vi "PH_ImageOperator.PC set Position On.vi"(0 "i ref in":refnum<vi>, 2 "Position on":bool, 5 "error in (no error)":errorcluster) -> (14 "i ref out":refnum<vi>, 19 "error out":errorcluster)   [LabVIEW 2014, in "PH_ImageOperator.lvlib"]
doc: "This is the Action of the \"PositionOn\"-Case: It sets some attributes and GUI elements."
uses:
  PH_ImageOperator.lvlib
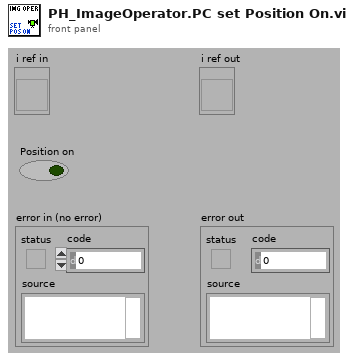
[diagram p1: front panel]
types:
  T1 = typedef "PH_ImageOperator.lvlib/PH_ImageOperator.i attribute.ctl" = cluster{"GUI Refs":cluster{"Delete":refnum<vi>, "Calibration status":refnum<vi>, "BI subtracted":refnum<vi>, "calc Energy":refnum<vi>, "Energy: expected value":refnum<vi>, "Energy: Tolerance":refnum<vi>, "Energy calculated":refnum<vi>, "Energy":refnum<vi>, "calc Beam Anal":refnum<vi>, "Maj Diam 1/esquare":refnum<vi>, "Min Diam 1/esquare":refnum<vi>, "Azi Angle":refnum<vi>, "Min/Maj Diam esquare":refnum<vi>, "Beam analysed":refnum<vi>, "CoG - x":refnum<vi>, "CoG - y":refnum<vi>, "BA: Method":refnum<vi>, "BA: Steps":refnum<vi>, "BA: Factor":refnum<vi>, "calc Traces":refnum<vi>, "Traces: Fit Gauss":refnum<vi>, "Traces calculated":refnum<vi>, "Maj FWHM":refnum<vi>, "Min FWHM":refnum<vi>, "Major Trace":refnum<vi>, "Minor Trace":refnum<vi>, "Maj Fit Order":refnum<vi>, "Min Fit Order":refnum<vi>, "Position calculated":refnum<vi>, "Position":refnum<vi>, "Type":refnum<vi>, "Center":refnum<vi>, "exp - X":refnum<vi>, "exp - Y":refnum<vi>, "Tolerance":refnum<vi>, "f":refnum<vi>, "M":refnum<vi>, "D":refnum<vi>, "q":refnum<vi>, "Dummy Method":refnum<vi>, "Dummy Type":refnum<vi>, "Global On":refnum<vi>, "Traces: No offset":refnum<vi>, "Maj 99%":refnum<vi>, "Min 99%":refnum<vi>, "GUI FF Image":refnum<vi>, "calc Fill Factor":refnum<vi>, "FF calculated":refnum<vi>, "Fill Factor: Filter?":refnum<vi>, "FF: Damage Threshold":refnum<vi>, "FF: Threshold":refnum<vi>, "FF: max allow. Energy":refnum<vi>, "FF: Fillfactor":refnum<vi>, "Calibration data":refnum<vi>}, "List of GUIs":string[], "Calibration":cluster{"Status":T2, "Calibration data":T3, "Calibration Data File":path}, "Final Image":cluster{"BI Subtraction Failure":bool}, "Energy":cluster{"on":bool, "expected value [mJ]":dbl, "Tolerance [%]":dbl, "State":T2, "Energy [mJ]":dbl, "Unit":string, "calculated @":timestamp}, "Beam Analysis":cluster{"on":bool, "Data":T4, "Method":bool, "Steps":i32, "Factor":i32, "ROI":cluster{"Left":i32, "Top":i32, "Right":i32, "Bottom":i32}, "analysed @":timestamp}, "Trace Analysis":cluster{"on":bool, "Fit on":bool, "Maj FWHM":dbl, "Min FWHM":dbl, "Maj Fit Order":i32, "Min Fit Order":i32, "No Offset":bool, "Maj 99%":dbl, "Min 99%":dbl, "Traces":cluster{"XScaleName":string, "Y Scale Minimum":sgl, "Y Scale Maximum":sgl, "X Scale Minimum":sgl, "X Scale Maximum":sgl, "Traces":cluster{"Index":sgl[], "Trace":dbl[]}[]}[], "analysed @":timestamp}, "Position Analysis":cluster{"on":bool, "exp - X":i32, "exp - Y":i32, "focal length [mm]":dbl, "Magnification":dbl, "Delta":dbl, "Theta":dbl, "Tolerance":dbl, "Type":bool, "analysed @":timestamp}, "Fill Factor":cluster{"on":bool, "Filter on?":bool, "Threshold":dbl, "Damage Threshold [J/cm²]":dbl, "Fillfactor":dbl, "Max. allowed Energy [J]":dbl, "calculated @":timestamp}, "Statistician Service ID":i32, "Images":cluster{"Background":T5, "OP":T5, "GUI":T5, "BA: ROI":T5, "Trace: Turn":T5, "FF: Main":T5, "FF: Help":T5, "PSDB: BG":T5, "PSDB: OP":T5, "PSDB: FF":T5}}
  T2 = typedef "PH_StatusHandler.lvlib/PH_StatusHandler.Status.ctl" = i16
  T3 = typedef "PH_ImageCalibrator.lvlib/PH_ImageCalibrator.Calibration Data.ctl" = cluster{"Date":string, "Time":string, "Cam Settings":cluster{"Cam ID":string, "Gain":dbl, "Brightness":dbl, "Shutter":dbl, "Cam Error":bool, "Mode":i32}, "Background Image":cluster{"Image":dbl[][], "Image Error":bool}, "Linear Calibration":cluster{"Calibration Factor":dbl, "not mm or mrad":bool}, "Energy Calibration":cluster{"Calibration Factor":dbl, "no mJ":bool}}
  T4 = typedef "PH_ImageOperator.lvlib/PH_ImageOperator.Beam Analysis Data.ctl" = cluster{"CoG-x":sgl, "CoG-y":sgl, "Maj Dim":dbl, "Min Dim":dbl, "Ellipticity":dbl, "Azimuth Angle [rad]":dbl, "Azi Angle rel to Maj?":bool}
  T5 = typedef "IMAQ Image.ctl" = refnum<image>
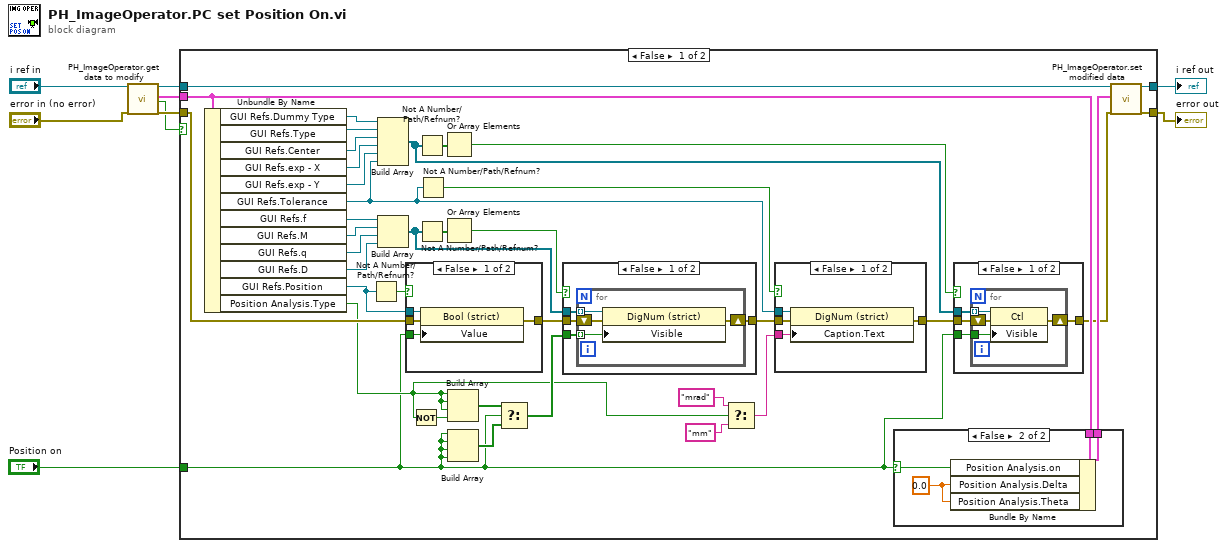
[diagram p0: block diagram]
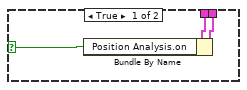
[diagram p2: hidden frame]
diagram:
  n1 = call "PH_ImageOperator.get data to modify.vi"("i ref in"="i ref in", "error in (no error)"="error in (no error)") -> ("i ref out"=w6:refnum<vi>, "i attribute"=w8:T1, "timed out"=w1:bool, "error out"=w4:errorcluster)  [unwired: 14 in]
  n2 = case shown="False" w1 {
    tunnel: "Position on" -> [w11 _]
    tunnel: w8 -> [w43 _]
    tunnel: [w46 w84] -> w7
    tunnel: w6 -> [w45 w84]
    tunnel: [w44 w83] -> w5
    tunnel: w4 -> [w42 w83]
    frame False {
      n3 = Unbundle By Name(w43) -> ("GUI Refs.Dummy Type"=w10:refnum<vi>, "GUI Refs.Type"=w36:refnum<vi>, "GUI Refs.Center"=w37:refnum<vi>, "GUI Refs.exp - X"=w38:refnum<vi>, "GUI Refs.exp - Y"=w39:refnum<vi>, "GUI Refs.Tolerance"=w17:refnum<vi>, "GUI Refs.f"=w29:refnum<vi>, "GUI Refs.M"=w28:refnum<vi>, "GUI Refs.q"=w27:refnum<vi>, "GUI Refs.D"=w26:refnum<vi>, "GUI Refs.Position"=w40:refnum<vi>, "Position Analysis.Type"=w15:bool)
      n4 = Not A Number/Path/Refnum?(number/path/refnum=w40) -> (NaN/Path/Refnum?=w41:bool)
      n5 = Build Array(w10, w36, w37, w38, w39, w17) -> (w32:refnum<vi>[])
      n6 = Build Array(w29, w28, w27, w26) -> (w25:refnum<vi>[])
      n7 = case shown="False" w41 {
        tunnel: w40 -> [w81 _]
        tunnel: w11 -> [w80 _]
        tunnel: w42 -> [w79 w82]
        tunnel: [w78 w82] -> w31
        frame False {
          n8 = property class="Bool (strict)"(reference=w81, error in=w79, "Value"=w80) -> (error out=w78:errorcluster)  [unwired: 1 out]
        }
        frame True {
        }
      }
      n9 = Not(x=w15) -> (.not. x?=w20:bool)
      n10 = Not A Number/Path/Refnum?(number/path/refnum=w32) -> (NaN/Path/Refnum?=w35:bool[])
      n11 = Not A Number/Path/Refnum?(number/path/refnum=w25) -> (NaN/Path/Refnum?=w30:bool[])
      n12 = Not A Number/Path/Refnum?(number/path/refnum=w17) -> (NaN/Path/Refnum?=w16:bool)
      n13 = Or Array Elements(Boolean array=w35) -> (logical OR=w33:bool)
      n14 = Or Array Elements(Boolean array=w30) -> (logical OR=w24:bool)
      n15 = Build Array(w15, w15, w15, w20) -> (w21:bool[])
      n16 = Build Array(w11, w11, w11, w11) -> (w23:bool[])
      n17 = Select(t=w21, s=w11, f=w23) -> (s? t:f=w22:bool[])
      n18 = case shown="False" w24 {
        tunnel: w25 -> [w63 _]
        tunnel: w22 -> [w62 _]
        tunnel: w31 -> [w61 w68]
        tunnel: [w60 w68] -> w19
        frame False {
          n19 = for {
            tunnel: w63 -> [w67] mode=indexing
            tunnel: w62 -> [w66] mode=indexing
            shift-right: [w64] -> w60
            shift-left: w61 -> [w65]
            n20 = property class="DigNum (strict)"(reference=w67, error in=w65, "Visible"=w66) -> (error out=w64:errorcluster)  [unwired: 1 out]
          }
        }
        frame True {
        }
      }
      n21 = Select(t="mrad", s=w15, f="mm") -> (s? t:f=w14:string)
      n22 = case shown="False" w16 {
        tunnel: w17 -> [w58 _]
        tunnel: w14 -> [w57 _]
        tunnel: w19 -> [w56 w59]
        tunnel: [w55 w59] -> w18
        frame False {
          n23 = property class="DigNum (strict)"(reference=w58, error in=w56, "Caption.Text"=w57) -> (error out=w55:errorcluster)  [unwired: 1 out]
        }
        frame True {
        }
      }
      n24 = case shown="False" w11 {
        selector: w11 -> [w48 w51]
        tunnel: [w50 w54] -> w47
        tunnel: w43 -> [w49 w53]
        frame True {
          n25 = Bundle By Name(cluster=w49, "Position Analysis.on"=w48) -> (w50:T1)
        }
        frame False {
          w52 = 0.0 ("Position Analysis.Delta")
          n26 = Bundle By Name(cluster=w53, "Position Analysis.on"=w51, "Position Analysis.Delta"=w52, "Position Analysis.Theta"=w52) -> (w54:T1)
        }
      }
      n27 = case shown="False" w33 {
        tunnel: w32 -> [w72 _]
        tunnel: w11 -> [w71 _]
        tunnel: w18 -> [w70 w77]
        tunnel: [w69 w77] -> w34
        frame False {
          n28 = for {
            tunnel: w72 -> [w76] mode=indexing
            tunnel: w71 -> [w75]
            shift-right: [w73] -> w69
            shift-left: w70 -> [w74]
            n29 = property class="Ctl"(reference=w76, error in=w74, "Visible"=w75) -> (error out=w73:errorcluster)  [unwired: 1 out]
          }
        }
        frame True {
        }
      }
      n30 = call "PH_ImageOperator.set modified data.vi"("i ref in"=w45, "i attribute"=w47, "error in (no error)"=w34) -> ("i ref out"=w46:refnum<vi>, "error out"=w44:errorcluster)  [unwired: 15 in]
    }
    frame True {
    }
  }
  "i ref out" <- w7
  "error out" <- w5
